vi "Inverse FHT.vi"(0 "X":dbl[](array[numeric])) -> (1 "Inv FHT {X}":dbl[](array[numeric]), 2 "error":i32)   [LabVIEW 2017, in "NI_AALPro.lvlib"]
doc: "Computes the inverse fast Hartley transform of the input sequence <B>X</B>."
uses:
  NI_AALPro.lvlib
  <resource>/lvanlys.dll
panel:
  # "Inverse Fast Hartley Transform"
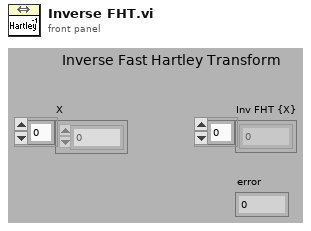
[diagram p1: front panel]
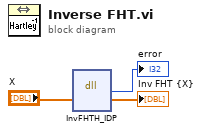
[diagram p0: block diagram]
diagram:
  n1 = dll-call lib="C:/Program Files (x86)/National Instruments/LabVIEW 2017/resource/lvanlys.*" fn="InvFHTH_IDP"("xH"="X") -> ("return type"=→"error":i32, "xH"=→"Inv FHT {X}":dbl[])  [unwired: 5 in, 2 out]
